vi "DS345.destructor.vi"(0 "i ref in":refnum<vi>, 5 "error in (no error)":errorcluster) -> (19 "error out":errorcluster)   [LabVIEW 2014, in "DS345.lvlib"]
doc: "This is the destructor of a class.\n\nLicense Agreement for this software:\n\nCopyright (C)\nGesellschaft für Schwerionenforschung, GSI\nPlanckstr. 1\n64291 Darmstadt\nGermany\n\nContact: D.Beck@gsi.de \n\nThis program is free software; you can redistribute it and/or modify it under the terms of the \nGNU General Public License as published by the Free Software Foundation; either version 2 of \nthe license, or (at your option) any later version.\n\nThis program is distributed in the hope that it will be useful, but WITHOUT ANY WARRANTY; \nwithout even the implied warranty of MERCHANTABILITY or FITNESS FOR A PARTICULAR PURPOSE. See the GNU General License for more details (http://www.gnu.org).\n\nGesellschaft für Schwerionenforschung, GSI\nPlanckstr. 1, 64291 Darmstadt, Germany\nFor all questions and ideas contact: M.Richter@gsi.de, H.Brand@gsi.de or D.Beck@gsi.de.\nLast update: 16-JUN-2004"
uses:
  DS345.lvlib
  CS_Core/CSApplicationBaseClasses/AFGBase/AFGBase.lvlib
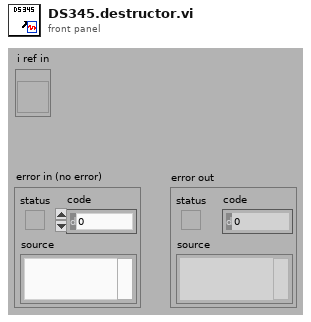
[diagram p1: front panel]
types:
  T1 = enum16{"SetAttribute", "GetAttribute", "CreateAttribute", "DestroyAttribute", "DestroyAllAtributes"}
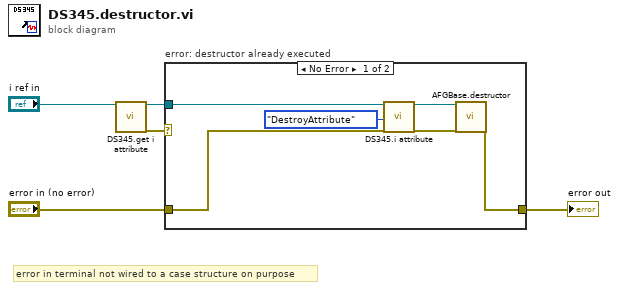
[diagram p0: block diagram]
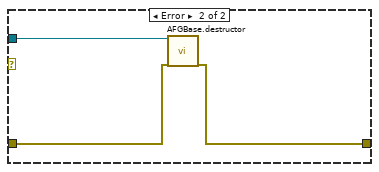
[diagram p2: hidden frame]
diagram:
  # "error in terminal not wired to a case structure on purpose"
  n1 = call "DS345.get i attribute.vi"("i ref in"="i ref in") -> ("i ref out"=w2:refnum<vi>, "error out"=w1:errorcluster)  [unwired: 16 in, 1 out]
  n2 = case "error: destructor already executed" shown="No Error" w1 {
    tunnel: [w9 w12] -> w5
    tunnel: "error in (no error)" -> [w7 w13]
    tunnel: w2 -> [w6 w14]
    frame No Error {
      n3 = call "DS345.i attribute.vi"("VI Refnum"=w6, "Action"=T1."DestroyAttribute", "error in (no error)"=w7) -> ("VI Refnum out"=w8:refnum<vi>, "error out"=w10:errorcluster)  [unwired: 14 in, 1 out]
      n4 = call "AFGBase.destructor.vi"("i ref in"=w8, "error in (no error)"=w10) -> ("error out"=w9:errorcluster)  [unwired: 17 in]
    }
    frame Error {
      n5 = call "AFGBase.destructor.vi"("i ref in"=w14, "error in (no error)"=w13) -> ("error out"=w12:errorcluster)  [unwired: 17 in]
    }
  }
  "error out" <- w5
